vi "LHF.DB.Mongo.Collection.FindVariant.vi"(8 "error in (no error)":errorcluster, 9 "query":refnum<k24>, 10 "Collection":string, 11 "LHF.DB.Mongo in":refnum<class "LHF.DB.Mongo.lvclass">) -> (0 "error out":errorcluster, 2 "Documents":variant[](array[variant]), 3 "LHF.DB.Mongo out":refnum<class "LHF.DB.Mongo.lvclass">, 5 "ObjectIDs":string[](array[string]))   [LabVIEW 2013, in "LHF.DB.Mongo.lvclass"]
uses:
  LHF.DB.Mongo.lvclass
  C:/Users/schim/Desktop/Projetos/LabVIEW-MongoDB/src/Driver/MongoDB.Driver.dll
  Driver/MongoDB.Driver.dll
panel:
  in  "type":variant
  in  "Extract _id":bool=TRUE
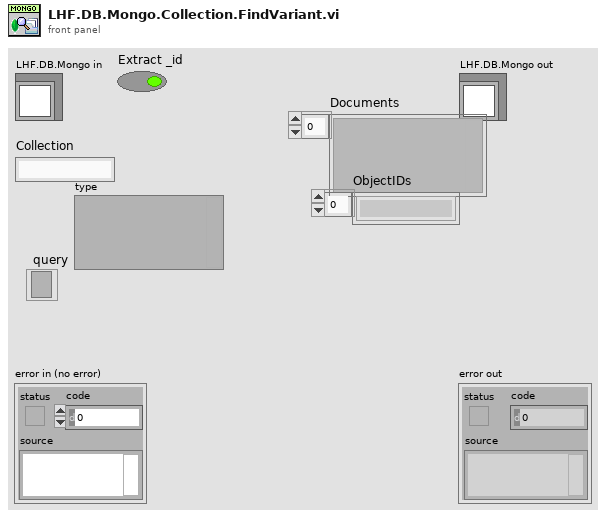
[diagram p1: front panel]
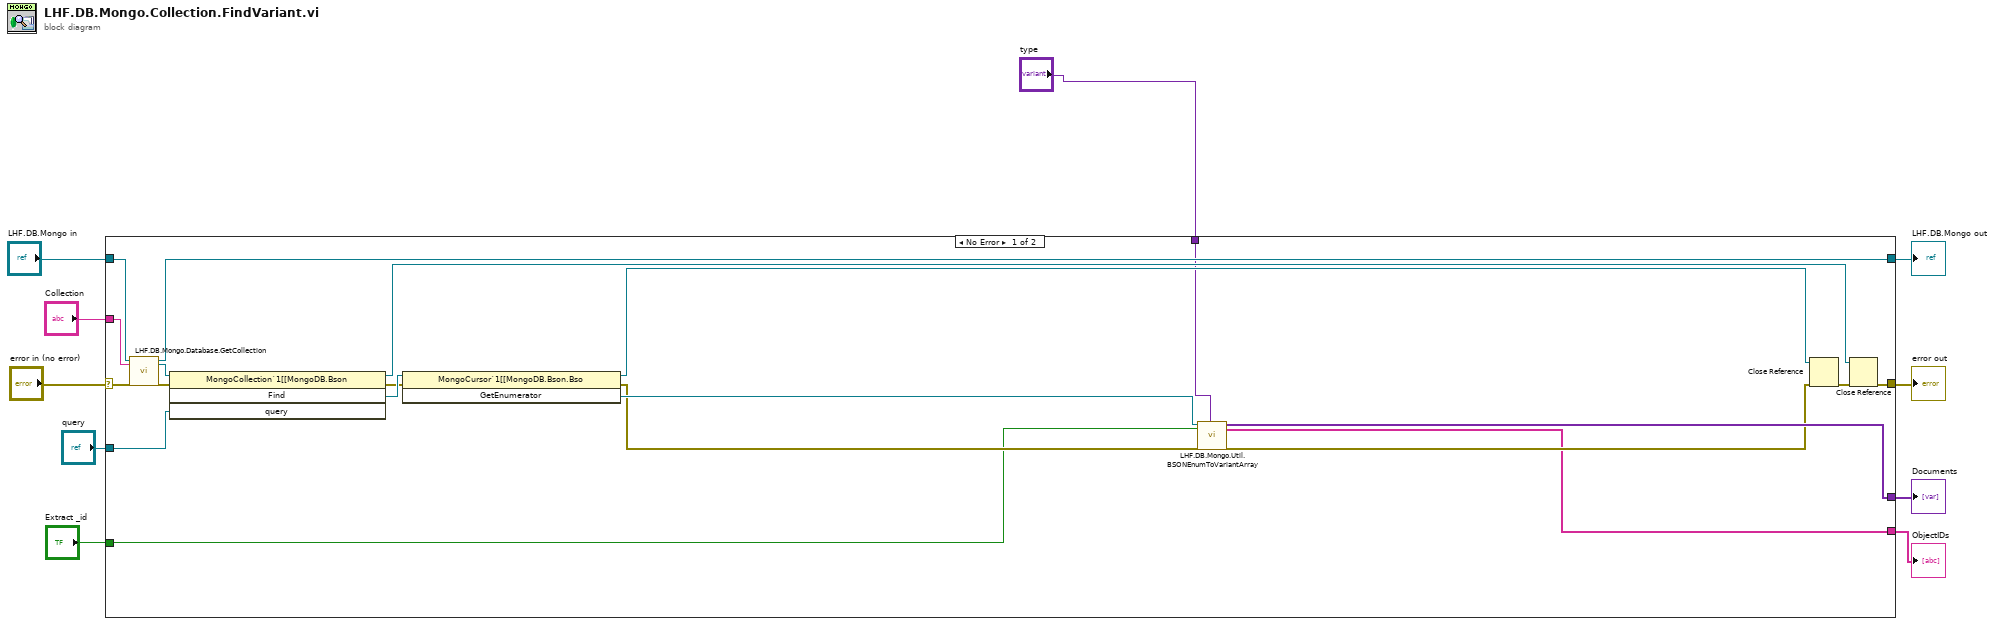
[diagram p0: block diagram]
diagram:
  n1 = case shown="No Error" "error in (no error)" {
    selector: "error in (no error)" -> [w16 w32]
    tunnel: [w19 w32] -> w9
    tunnel: [w29 w31] -> w7
    tunnel: "LHF.DB.Mongo in" -> [w28 w31]
    tunnel: "Collection" -> [w30 _]
    tunnel: [w25 _] -> w5
    tunnel: "query" -> [w15 _]
    tunnel: [w13 _] -> w3
    tunnel: "Extract _id" -> [w12 _]
    tunnel: "type" -> [w11 _]
    frame No Error {
      n2 = call "LHF.DB.Mongo.Database.GetCollection.vi"("LHF.DB.Mongo in"=w28, "collectionName"=w30, "error in (no error)"=w16) -> ("LHF.DB.Mongo in"=w29:refnum<class "LHF.DB.Mongo.lvclass">, "MongoCollection"=w17:refnum<k24>, "error out"=w14:errorcluster)  [unwired: 14 in]
      n3 = invoke class="MongoCollection`1[[MongoDB.Bson" method="Find"(reference=w17, error in=w14, "query"=w15) -> (reference out=w21:refnum<k24>, error out=w23:errorcluster, "Find"=w27:refnum<k24>)  [unwired: 1 in, 1 out]
      n4 = invoke class="MongoCursor`1[[MongoDB.Bson.Bso" method="GetEnumerator"(reference=w27, error in=w23) -> (reference out=w22:refnum<k24>, error out=w24:errorcluster, "GetEnumerator"=w26:refnum<k24>)  [unwired: 1 in]
      n5 = call "LHF.DB.Mongo.Util.BSONEnumToVariantArray.vi"("BsonENUM"=w26, "Extract ObjectID"=w12, "error in (no error)"=w24, "type"=w11) -> ("Documents"=w25:variant[], "ObjectIDs"=w13:string[], "error out"=w18:errorcluster)  [unwired: 13 in]
      n6 = Close Reference(reference=w22, error in (no error)=w18) -> (error out=w20:errorcluster)
      n7 = Close Reference(reference=w21, error in (no error)=w20) -> (error out=w19:errorcluster)
    }
    frame Error {
    }
  }
  "error out" <- w9
  "LHF.DB.Mongo out" <- w7
  "Documents" <- w5
  "ObjectIDs" <- w3
